vi "New_GraphDisp.vi"() -> ()   [LabVIEW 2016, in "PanelSplitForDisplay.lvclass"]
uses:
  PanelSplit/PanelSplitForDisplay.lvclass
  PanelSplit/PanelObject/PanelObject.lvclass
  <vilib>/Utility/error.llb/DialogType.ctl
  PanelSplit/PanelDataNode/PanelDataNode.lvclass
  Architecture/Queue Management/ARC_Queue Create_Single.vi
  Architecture/Queue Management/ARC_Queue Remove Element.vi
  Ctrls/GlobeVaribles.vi
  Architecture/Queue Management/ARC_Queue Insert Element.vi
  Architecture/Queue Management/ARC_Queue Destroy_Single.vi
panel:
  in  "Node*":refnum<data-value>
  out "Waveform Chart":waveform(dbl)(graph)
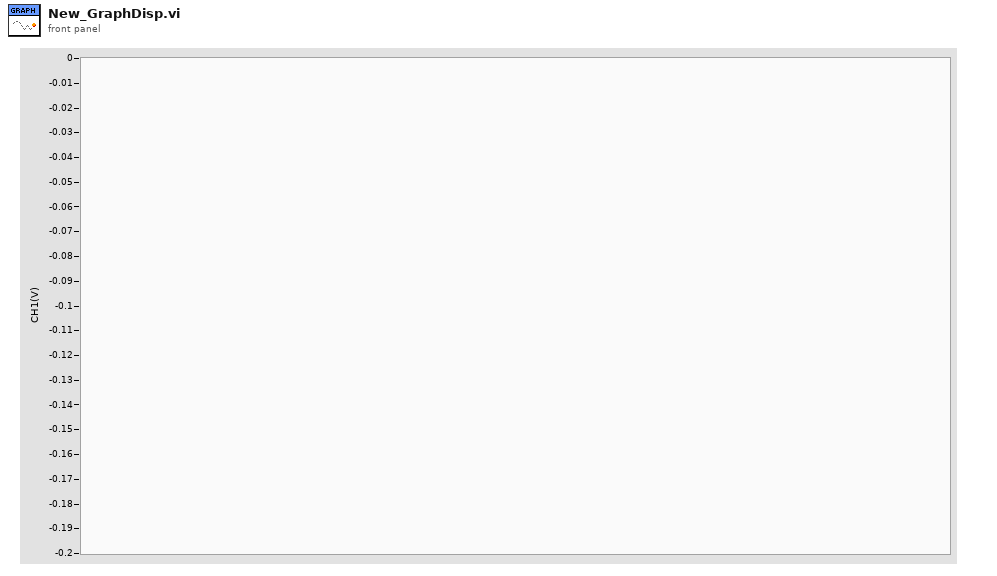
[diagram p1: front panel]
types:
  T1 = cluster{"error":errorcluster, "Event":string, "Data":variant, "Q_Local":string, "Graph":refnum<vi>, "Q_Caller":string}
  T2 = typedef "DialogType.ctl" = u16
  T3 = typedef "LVRectTypeDef.ctl" = cluster{"Left":i16, "Top":i16, "Right":i16, "Bottom":i16}
  T4 = typedef "PanelSplitForDisplay.lvclass/ViValueCtl.ctl" = cluster{"CHTag":string, "GraphProperts":cluster{"YMax":dbl, "YMin":dbl, "ScaleFit":u8}, "CHUnit":string, "CHName":string, "CHValue":string, "CHAlias":string}
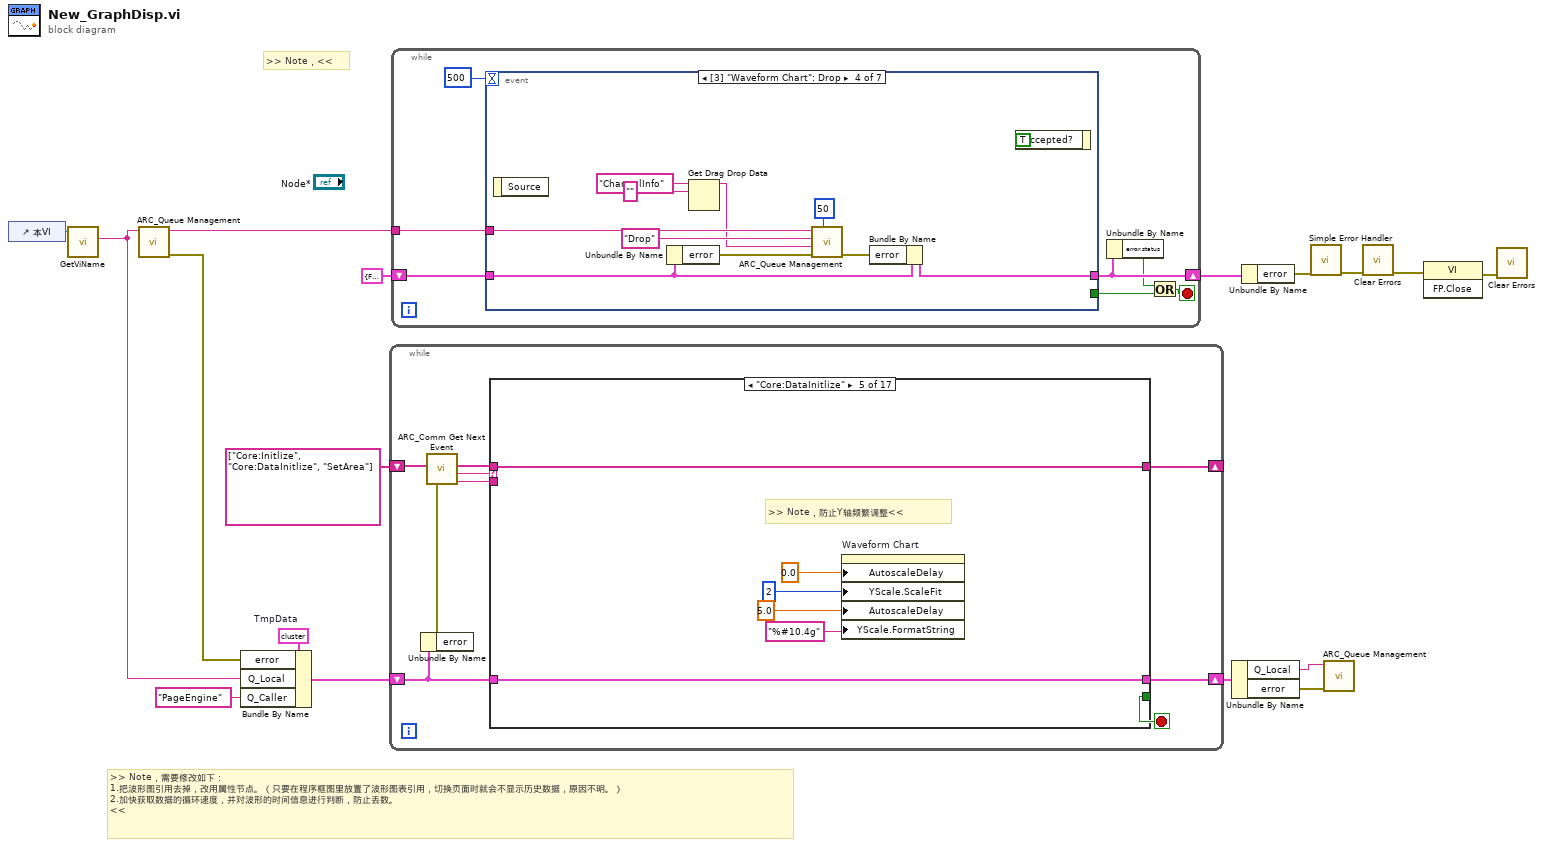
[diagram p0: block diagram]
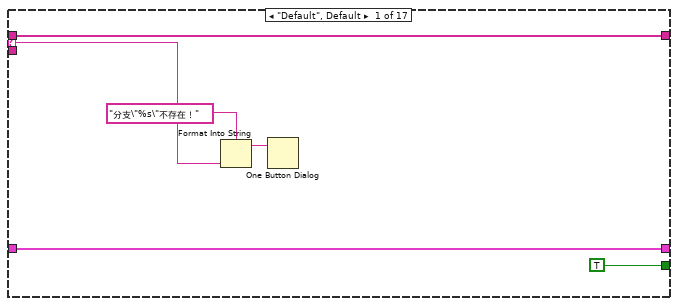
[diagram p2: hidden frame]
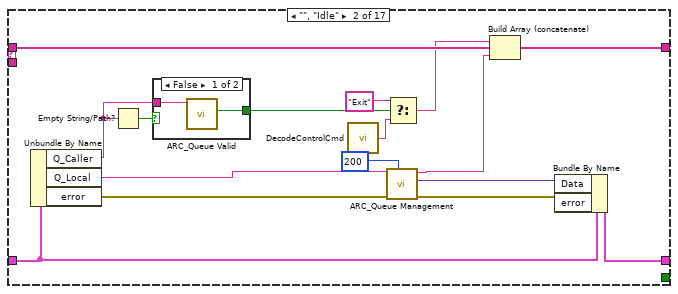
[diagram p3: hidden frame]
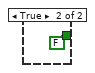
[diagram p4: hidden frame]
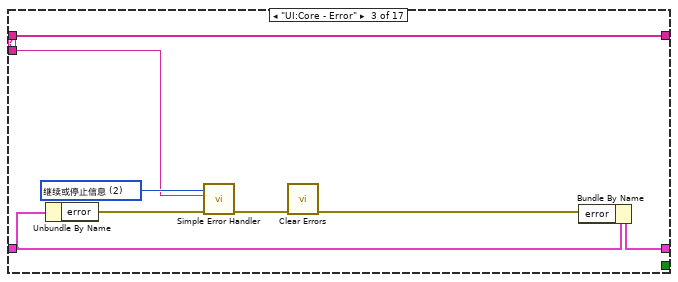
[diagram p5: hidden frame]
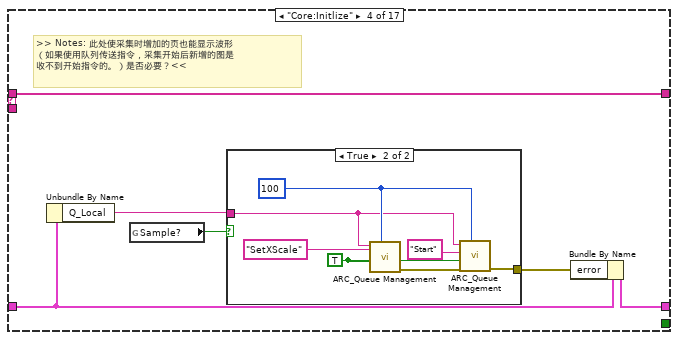
[diagram p6: hidden frame]
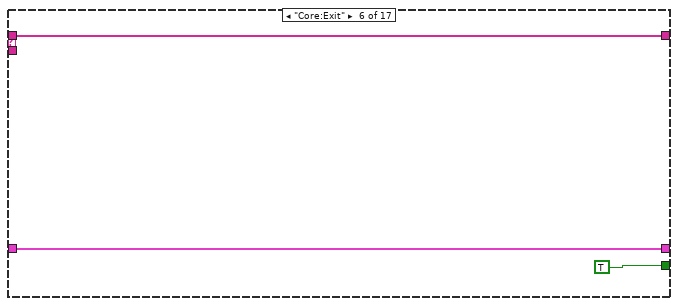
[diagram p8: hidden frame]
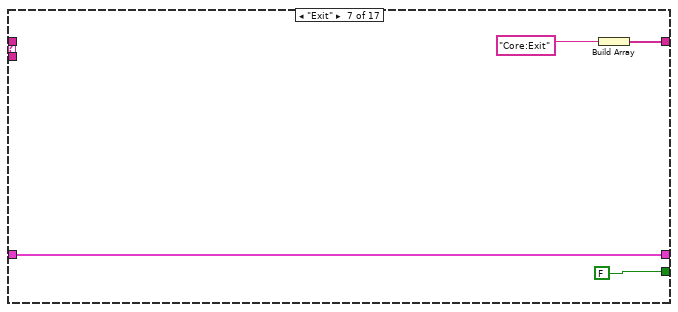
[diagram p9: hidden frame]
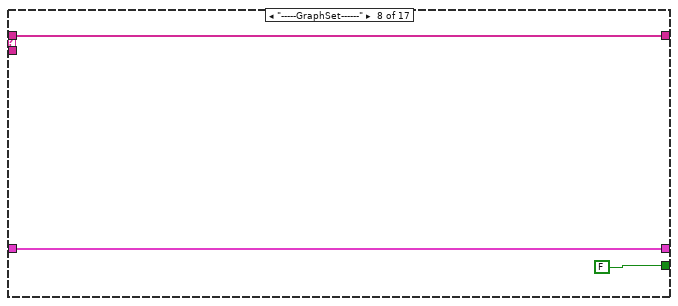
[diagram p10: hidden frame]
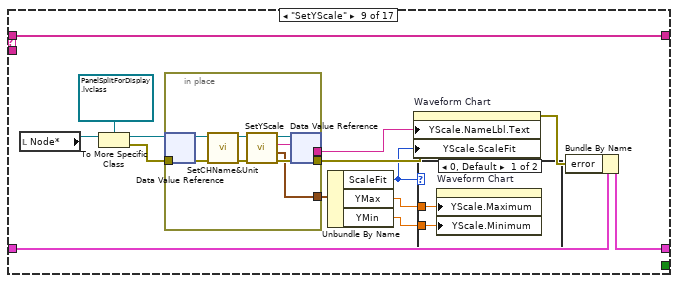
[diagram p11: hidden frame]
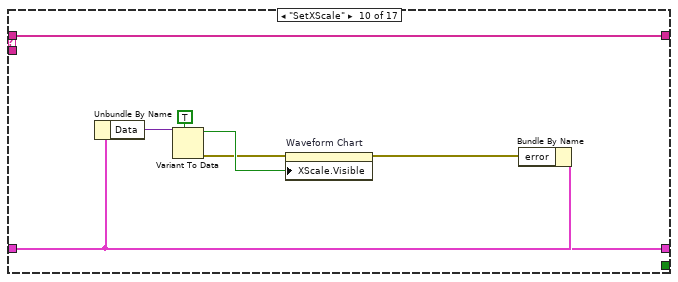
[diagram p13: hidden frame]
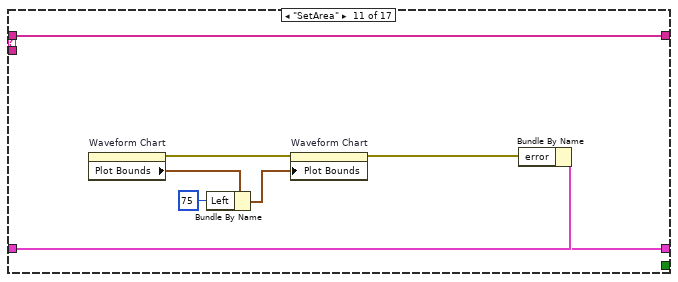
[diagram p14: hidden frame]
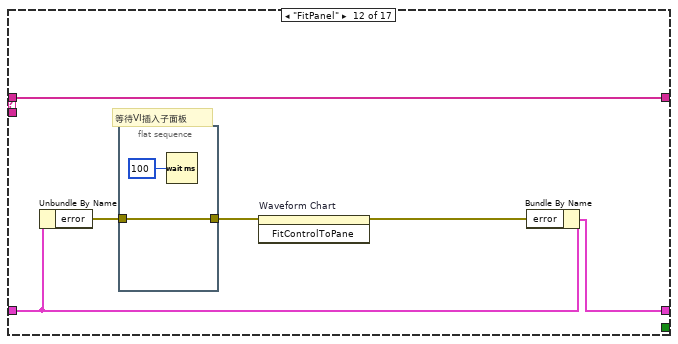
[diagram p15: hidden frame]
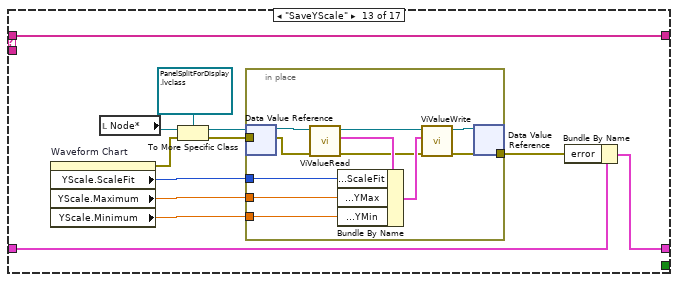
[diagram p16: hidden frame]
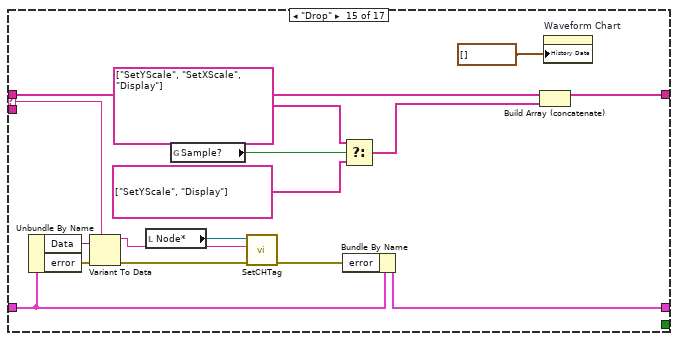
[diagram p18: hidden frame]
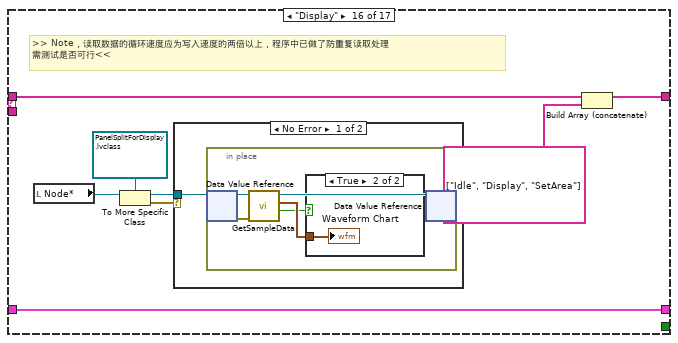
[diagram p19: hidden frame]
diagram:
  w14 = T1 {"error"={"status"=FALSE, "code"=0, "source"=""}, "Event"="", "Data"=variant, "Q_Local"="", "Graph"=refnum, "Q_Caller"=""}  # TmpData
  # ">> Note，<<"
  # ">> Note，需要修改如下：\n1.把波形图引用去掉，改用属性节点。（只要在程序框图里放置了波形图表引用，切换页面时就会不显示历史数据，原因不明。）\n2.加快获取数据的循环速度，并对波形的时间信息进行判断，防止丢数。\n<<"
  n1 = control-ref of="本VI"() -> (w7:refnum<vi>)
  n2 = call "GetViName.vi"("VI*"=w7) -> ("VI Name"=w10:string)  [unwired: 9 in, 1 out]
  n3 = call-poly "ARC_Queue Management.vi"("Queue Name"=w10) -> ("error out"=w11:errorcluster)  [unwired: 8 in, 2 out]
  n4 = Bundle By Name(cluster=w14, "error"=w11, "Q_Local"=w10, "Q_Caller"="PageEngine") -> (w13:T1)
  n5 = while {
    shift-right: [w21] -> w15
    shift-left: w13 -> [w22]
    shift-right: [w20] -> _
    shift-left: string[] ["Core:Initlize", "Core:DataInitlize", "SetArea"] ("event queue out") -> [w19]
    stop <- w24 stop-if-true
    n6 = Unbundle By Name(w22) -> ("error"=w23:errorcluster)
    n7 = call "ARC_Comm Get Next Event.vi"("error in (no error)"=w23, "event queue in"=w19) -> ("prev event"=w25:string, "next event"=w17:string, "event queue out"=w18:string[])  [unwired: 4 in]
    n8 = case shown="\"Core:DataInitlize\"" w17 {
      selector: w17 -> [w29 _ _ _ _ _ _ _ _ _ _ _ _ _ w164 _ _]
      tunnel: w18 -> [w30 w36 w58 w59 w77 w78 _ w85 w101 w119 w127 w133 w147 w159 w175 w179 w192]
      tunnel: w25 -> [_ _ w51 _ _ _ _ _ _ _ _ _ _ _ _ _ _]
      tunnel: [TRUE _ _ _ _ TRUE FALSE FALSE _ _ _ _ _ _ _ _ _] -> w24
      tunnel: w22 -> [w31 w44 w54 w63 w76 w79 w83 w86 w94 w116 w126 w129 w138 w160 w172 w184 w193]
      tunnel: [w31 w46 w53 w64 w76 w79 w83 w86 w93 w115 w125 w131 w137 w160 w162 w184 w193] -> w21
      tunnel: [w30 w35 w58 w59 w77 w78 w81 w85 w101 w119 w127 w133 w147 w159 w174 w178 w192] -> w20
      frame "Default", Default {
        n9 = Format Into String(format string="分支\"%s\"不存在！" ("格式字符串"), w29) -> (resulting string=w28:string)  [unwired: 2 in, 1 out]
        n10 = One Button Dialog(message=w28) -> ()  [unwired: 1 in, 1 out]
      }
      frame "", "Idle" {
        n11 = Unbundle By Name(w44) -> ("Q_Caller"=w39:string, "Q_Local"=w43:string, "error"=w37:errorcluster)
        n12 = Empty String/Path?(string/path=w39) -> (empty?=w40:bool)
        n13 = case shown="False" w40 {
          tunnel: [w48 FALSE ("Not Exist?")] -> w38
          tunnel: w39 -> [w49 _]
          frame False {
            n14 = call "ARC_Queue Valid.vi"("Queue Name(unamed)"=w49) -> ("Not Exist?"=w48:bool)  [unwired: 8 in, 2 out]
          }
          frame True {
          }
        }
        n15 = call "DecodeControlCmd.vi"() -> ("Command"=w41:string)
        n16 = call-poly "ARC_Queue Management.vi"("Time out(-1)_queue out"=200 ("Time out(-1)"), "error in (no error)"=w37, "Queue Name(unamed)"=w43) -> ("error out"=w47:errorcluster, "Data"=w45:variant, "Event"=w33:string)  [unwired: 5 in, 1 out]
        n17 = Select(t="Exit" ("Event"), s=w38, f=w41) -> (s? t:f=w34:string)
        n18 = Build Array (concatenate)(w34, w36, w33) -> (w35:string[])
        n19 = Bundle By Name(cluster=w44, "Data"=w45, "error"=w47) -> (w46:T1)
      }
      frame "UI:Core - Error" {
        w52 = T2 2 items=["无对话框", "确定信息", "继续或停止信息", "确定信息＋警告", "继续/停止+警告"] ("type of dialog (OK msg:1)")
        n20 = Unbundle By Name(w54) -> ("error"=w55:errorcluster)
        n21 = call <vilib>:"Simple Error Handler.vi"("error source (\" \")"=w51, "type of dialog (OK msg:1)"=w52, "error in (no error)"=w55) -> ("error out"=w56:errorcluster)  [unwired: 2 in, 4 out]
        n22 = call <vilib>:"Clear Errors.vi"("error in (no error)"=w56) -> ("error out"=w57:errorcluster)  [unwired: 5 in, 1 out]
        n23 = Bundle By Name(cluster=w54, "error"=w57) -> (w53:T1)
      }
      frame "Core:Initlize" {
        # ">> Notes: 此处使采集时增加的页也能显示波形\n（如果使用队列传送指令，采集开始后新增的图是\n收不到开始指令的。）是否必要？<<"
        n24 = Unbundle By Name(w63) -> ("Q_Local"=w62:string)
        n25 = global read "GlobeVaribles.vi" "Sample?"() -> (w60:bool)
        n26 = case shown="True" w60 {
          tunnel: w62 -> [_ w67]
          tunnel: [_ w69] -> w61
          frame False {
          }
          frame True {
            w68 = 100 ("Time out(-1)_queue in")
            w65 = TRUE
            n27 = call-poly "ARC_Queue Management.vi"("Time out(-1)_queue in"=w68, "Data"=w65, "Event"="SetXScale", "Queue Name(unamed)"=w67) -> ("error out"=w70:errorcluster)  [unwired: 6 in, 1 out]
            n28 = call-poly "ARC_Queue Management.vi"("Time out(-1)_queue in"=w68, "error in (no error)"=w70, "Data"=w65, "Event"="Start", "Queue Name(unamed)"=w67) -> ("error out"=w69:errorcluster)  [unwired: 5 in, 1 out]
          }
        }
        n29 = Bundle By Name(cluster=w63, "error"=w61) -> (w64:T1)
      }
      frame "Core:DataInitlize" {
        # ">> Note，防止Y轴频繁调整<<"
        n30 = property on="Waveform Chart" class="WFChart (strict)"("AutoscaleDelay"=sgl 0.0 ("自动调整标尺延迟"), "YScale.ScaleFit"=u8 2 ("Y标尺.标尺调节"), "AutoscaleDelay"=sgl 5.0 ("自动调整标尺延迟"), "YScale.FormatString"="%#10.4g" ("Y标尺.格式字符串")) -> ()  [unwired: 2 in, 2 out]
      }
      frame "Core:Exit" {
      }
      frame "Exit" {
        n31 = Build Array("Core:Exit" ("Remaining States")) -> (w81:string[])
      }
      frame "-----GraphSet------" {
      }
      frame "SetYScale" {
        n32 = local read "Node*"() -> (w100:refnum<data-value>)
        n33 = To More Specific Class(target class=refnum<data-value> refnum ("数据值引用"), reference=w100) -> (specific class reference=w99:refnum<data-value>, error out=w97:errorcluster)  [unwired: 1 in]
        n34 = in-place {
          in-place-border: w97 -> [w106]
          in-place-border: [w110] -> w96
          in-place-border: [w109] -> w95
          in-place-border: [w104] -> w92
          n35 = in-place-dvr #1(w99) -> (w108:refnum<class "PanelSplitForDisplay.lvclass">)  [unwired: 1 out]
          n36 = call "SetCHName&Unit.vi"("error in (no error)"=w106, "PanelSplitForDisplay 输入"=w108) -> ("error out"=w105:errorcluster, "PanelSplitForDisplay 输出"=w107:refnum<class "PanelSplitForDisplay.lvclass">)  [unwired: 8 in]
          n37 = call "SetYScale.vi"("error in"=w105, "PanelSplitForDisplay 输入"=w107) -> ("error out"=w109:errorcluster, "GraphProperts"=w104:cluster{"YMax":dbl, "YMin":dbl, "ScaleFit":u8}, "YLable"=w110:string, "PanelSplitForDisplay 输出"=w111:refnum<class "PanelSplitForDisplay.lvclass">)  [unwired: 6 in]
          n38 = in-place-dvr #1(w111) -> ()  [unwired: 2 out]
        }
        n39 = Unbundle By Name(w92) -> ("ScaleFit"=w91:u8, "YMax"=w90:dbl, "YMin"=w89:dbl)
        n40 = property on="Waveform Chart" class="WFChart (strict)"(error in=w95, "YScale.NameLbl.Text"=w96, "YScale.ScaleFit"=w91) -> (error out=w88:errorcluster)  [unwired: 1 in, 1 out]
        n41 = case shown="0, Default" w91 {
          tunnel: w90 -> [w103 _]
          tunnel: w89 -> [w102 _]
          frame 0, Default {
            n42 = property on="Waveform Chart" class="WFChart (strict)"("YScale.Maximum"=w103, "YScale.Minimum"=w102) -> ()  [unwired: 2 in, 2 out]
          }
          frame 2 {
          }
        }
        n43 = Bundle By Name(cluster=w94, "error"=w88) -> (w93:T1)
      }
      frame "SetXScale" {
        n44 = Unbundle By Name(w116) -> ("Data"=w117:variant)
        n45 = Variant To Data(type=TRUE ("X标尺.可见"), Variant=w117) -> (data=w114:bool, error out=w113:errorcluster)  [unwired: 1 in]
        n46 = property on="Waveform Chart" class="WFChart (strict)"(error in=w113, "XScale.Visible"=w114) -> (error out=w112:errorcluster)  [unwired: 1 in, 1 out]
        n47 = Bundle By Name(cluster=w116, "error"=w112) -> (w115:T1)
      }
      frame "SetArea" {
        n48 = property on="Waveform Chart" class="WFChart (strict)"() -> (error out=w120:errorcluster, "Plot Bounds"=w123:T3)  [unwired: 2 in, 1 out]
        n49 = Bundle By Name(cluster=w123, "Left"=i16 75 ("left")) -> (w122:T3)
        n50 = property on="Waveform Chart" class="WFChart (strict)"(error in=w120, "Plot Bounds"=w122) -> (error out=w124:errorcluster)  [unwired: 1 in, 1 out]
        n51 = Bundle By Name(cluster=w126, "error"=w124) -> (w125:T1)
      }
      frame "FitPanel" {
        # "等待VI插入子面板"
        n52 = Unbundle By Name(w129) -> ("error"=w128:errorcluster)
        n53 = flat-sequence {
          tunnel: [w134] -> w130
          tunnel: w128 -> [w134]
          frame #0 {
            n54 = Wait (ms)(milliseconds to wait=u32 100 ("等待时间（毫秒）")) -> ()  [unwired: 1 out]
          }
        }
        n55 = invoke on="Waveform Chart" class="WFChart (严格)" method="FitControlToPane"(error in=w130) -> (error out=w132:errorcluster)  [unwired: 2 in, 2 out]
        n56 = Bundle By Name(cluster=w129, "error"=w132) -> (w131:T1)
      }
      frame "SaveYScale" {
        n57 = property on="Waveform Chart" class="WFChart (strict)"() -> (error out=w136:errorcluster, "YScale.ScaleFit"=w142:u8, "YScale.Maximum"=w141:dbl, "YScale.Minimum"=w140:dbl)  [unwired: 2 in, 1 out]
        n58 = local read "Node*"() -> (w146:refnum<data-value>)
        n59 = To More Specific Class(target class=refnum<data-value> refnum ("数据值引用"), reference=w146, error in=w136) -> (specific class reference=w143:refnum<data-value>, error out=w144:errorcluster)
        n60 = in-place {
          in-place-border: w144 -> [w150]
          in-place-border: w142 -> [w153]
          in-place-border: w141 -> [w152]
          in-place-border: w140 -> [w151]
          in-place-border: [w148] -> w139
          n61 = in-place-dvr #2(w143) -> (w158:refnum<class "PanelSplitForDisplay.lvclass">)  [unwired: 1 out]
          n62 = call "ViValueRead.vi"("error in (no error)"=w150, "PanelSplitForDisplay 输入"=w158) -> ("error out"=w149:errorcluster, "ViValue"=w155:T4, "PanelSplitForDisplay 输出"=w157:refnum<class "PanelSplitForDisplay.lvclass">)  [unwired: 7 in]
          n63 = Bundle By Name(cluster=w155, "GraphProperts.ScaleFit"=w153, "GraphProperts.YMax"=w152, "GraphProperts.YMin"=w151) -> (w154:T4)
          n64 = call "ViValueWrite.vi"("error in (no error)"=w149, "ViValue"=w154, "PanelSplitForDisplay 输入"=w157) -> ("error out"=w148:errorcluster, "PanelSplitForDisplay 输出"=w156:refnum<class "PanelSplitForDisplay.lvclass">)  [unwired: 7 in]
          n65 = in-place-dvr #2(w156) -> ()  [unwired: 2 out]
        }
        n66 = Bundle By Name(cluster=w138, "error"=w139) -> (w137:T1)
      }
      frame "----------------------" {
      }
      frame "Drop" {
        n67 = Unbundle By Name(w172) -> ("Data"=w165:variant, "error"=w167:errorcluster)
        n68 = Variant To Data(error in=w167, type=w164, Variant=w165) -> (data=w163:string, error out=w166:errorcluster)
        n69 = local read "Node*"() -> (w173:refnum<data-value>)
        n70 = global read "GlobeVaribles.vi" "Sample?"() -> (w171:bool)
        n71 = call "SetCHTag.vi"("error in (no error)"=w166, "ChannelTag"=w163, "Node*"=w173) -> ("error out"=w161:errorcluster)  [unwired: 8 in]
        n72 = Bundle By Name(cluster=w172, "error"=w161) -> (w162:T1)
        n73 = Select(t=string[] ["SetYScale", "SetXScale", "Display"] ("event queue out"), s=w171, f=string[] ["SetYScale", "Display"] ("event queue out")) -> (s? t:f=w168:string[])
        n74 = Build Array (concatenate)(w175, w168) -> (w174:string[])
        n75 = property on="Waveform Chart" class="WFChart (strict)"("History Data"=waveform(dbl)[] [] ("历史数据")) -> ()  [unwired: 2 in, 2 out]
      }
      frame "Display" {
        # ">> Note，读取数据的循环速度应为写入速度的两倍以上，程序中已做了防重复读取处理\n需测试是否可行<<"
        n76 = local read "Node*"() -> (w183:refnum<data-value>)
        n77 = To More Specific Class(target class=refnum<data-value> refnum ("数据值引用"), reference=w183) -> (specific class reference=w182:refnum<data-value>, error out=w180:errorcluster)  [unwired: 1 in]
        n78 = case shown="No Error" w180 {
          tunnel: w182 -> [w185 _]
          frame No Error {
            n79 = in-place {
              n80 = in-place-dvr #3(w185) -> (w190:refnum<class "PanelSplitForDisplay.lvclass">, w187:errorcluster)
              n81 = call "GetSampleData.vi"("error in"=w187, "PanelSplitForDisplay.lvclass"=w190) -> ("Display?"=w186:bool, "signal out"=w188:waveform(dbl), "PanelSplitForDisplay.lvclass 2"=w189:refnum<class "PanelSplitForDisplay.lvclass">)  [unwired: 3 in, 2 out]
              n82 = case shown="True" w186 {
                tunnel: w188 -> [_ w191]
                frame False {
                }
                frame True {
                  "Waveform Chart" <- w191
                }
              }
              n83 = in-place-dvr #3(w189) -> ()  [unwired: 2 out]
            }
          }
          frame Error {
          }
        }
        n84 = Build Array (concatenate)(w179, string[] ["Idle", "Display", "SetArea"] ("event queue out")) -> (w178:string[])
      }
      frame "Stop" {
      }
    }
  }
  n85 = while {
    tunnel: w10 -> [w200]
    shift-right: [w195] -> w8
    shift-left: cluster{"Float?":bool, "error":errorcluster} {"Float?"=FALSE, "error"={"status"=FALSE, "code"=0, "source"=""}} -> [w199]
    stop <- w197 stop-if-true
    n86 = event shown="[3] \"Waveform Chart\": Drop" {
      selector: _ -> [_ _ _ _ _ _ _]
      dyn-events: _ -> [_ _ _ _ _ _ _]
      timeout: 500 -> [_ _ _ _ _ _ _]
      tunnel: [w201 _ _ _ _ _ FALSE] -> w198
      tunnel: w200 -> [w204 _ w218 w259 _ w266 _]
      tunnel: w199 -> [w202 w211 w220 w257 w262 w267 w270]
      tunnel: [w202 w211 w219 w255 w262 w267 w269] -> w195
      event Timeout {
        n87 = event-data() -> ()  [unwired: 1 in, 2 out]
        n88 = Unbundle By Name(w202) -> ("error"=w203:errorcluster)
        n89 = call-poly "ARC_Queue Management.vi"("error in"=w203, "Queue Name"=w204) -> ("Created New?"=w201:bool)  [unwired: 7 in, 2 out]
      }
      event "Waveform Chart": Shortcut Menu Activation? {
        w205 = string[] ["显示", "隐藏"] ("f")
        n90 = event-data() -> ("MenuRef"=w215:refnum<k9>)  [unwired: 1 in]
        n91 = Unbundle By Name(w211) -> ("Float?"=w210:bool)
        n92 = Not(x=w210) -> (.not. x?=w209:bool)
        n93 = Select(t=string[] ["删除", "浮动", "时间轴", "自动调整Y标尺"] ("项名称"), s=w209, f=string[] ["返回", "时间轴"]) -> (s? t:f=w213:string[])
        n94 = Delete Menu Items(9:w215) -> (0:w216:errorcluster, 3:w217:refnum<k9>)  [unwired: 3 in]
        n95 = Insert Menu Items(6:w216, 7:w213, 8:w213, 9:w217) -> (0:w207:errorcluster, 3:w208:refnum<k9>)  [unwired: 2 in, 1 out]
        n96 = Insert Menu Items(5:"时间轴", 6:w207, 7:w205, 8:w205, 9:w208) -> ()  [unwired: 1 in, 3 out]
        n97 = event-data() -> ()  [unwired: 2 in, 1 out]
      }
      event "Waveform Chart": Shortcut Menu Selection (User) {
        n98 = event-data() -> ("ItemTag"=w222:string)  [unwired: 1 in]
        n99 = local read "Node*"() -> (w223:refnum<data-value>)
        n100 = To More Specific Class(target class=refnum<data-value> refnum ("Node*"), reference=w223) -> (specific class reference=w221:refnum<data-value>)  [unwired: 1 in, 1 out]
        n101 = case shown="\"浮动\"" w222 {
          tunnel: w221 -> [_ w227 w231 w238 _ _ _ _]
          tunnel: w220 -> [w225 w226 w230 w237 w243 w245 w246 w250]
          tunnel: [w225 w226 w229 w235 w243 w245 w246 w250] -> w219
          tunnel: w218 -> [_ _ _ _ _ _ _ w247]
          frame "假", Default {
          }
          frame "删除" {
            n102 = call "Q_Delete.vi"("ChildNode*"=w227) -> ()  [unwired: 10 in, 1 out]
          }
          frame "浮动" {
            n103 = in-place {
              n104 = in-place-dvr #4(w231) -> (w234:refnum<class "PanelDataNode.lvclass">, w232:errorcluster)
              n105 = call "RefreshPanel.vi"("error in (no error)"=w232, "PanelDataNode 输入"=w234) -> ("PanelDataNode 输出"=w233:refnum<class "PanelDataNode.lvclass">)  [unwired: 8 in, 1 out]
              n106 = in-place-dvr #4(w233) -> ()  [unwired: 2 out]
            }
            n107 = Bundle By Name(cluster=w230, "Float?"=TRUE) -> (w229:cluster{"Float?":bool, "error":errorcluster})
          }
          frame "返回" {
            n108 = in-place {
              n109 = in-place-dvr #5(w238) -> (w241:refnum<class "PanelDataNode.lvclass">, w239:errorcluster)
              n110 = call "BackToPanel.vi"("error in (no error)"=w239, "PanelDataNode 输入"=w241) -> ("PanelDataNode 输出"=w240:refnum<class "PanelDataNode.lvclass">)  [unwired: 8 in, 1 out]
              n111 = in-place-dvr #5(w240) -> ()  [unwired: 2 out]
            }
            n112 = Bundle By Name(cluster=w237, "Float?"=FALSE) -> (w235:cluster{"Float?":bool, "error":errorcluster})
          }
          frame "显示" {
            n113 = property on="Waveform Chart" class="WFChart (strict)"("XScale.Visible"=TRUE ("X标尺.可见")) -> ()  [unwired: 2 in, 2 out]
          }
          frame "隐藏" {
            n114 = property on="Waveform Chart" class="WFChart (strict)"("XScale.Visible"=FALSE ("X标尺.可见")) -> ()  [unwired: 2 in, 2 out]
          }
          frame "Fit" {
            n115 = invoke on="Waveform Chart" class="WFChart (严格)" method="FitControlToPane"() -> ()  [unwired: 3 in, 3 out]
          }
          frame "自动调整Y标尺" {
            n116 = property on="Waveform Chart" class="WFChart (strict)"("YScale.ScaleFit"=u8 2 ("Y标尺.标尺调节")) -> ()  [unwired: 2 in, 2 out]
            n117 = call-poly "ARC_Queue Management.vi"("Event"="SaveYScale", "Queue Name(unamed)"=w247) -> ()  [unwired: 8 in, 2 out]
          }
        }
      }
      event "Waveform Chart": Drop {
        n118 = event-data() -> ()  [unwired: 1 in, 1 out]
        n119 = Unbundle By Name(w257) -> ("error"=w256:errorcluster)
        n120 = Get Drag Drop Data(8:"", 9:"ChannelInfo" ("数据名称")) -> (3:w251:string)  [unwired: 1 in, 1 out]
        n121 = call-poly "ARC_Queue Management.vi"("Time out(-1)_queue in"=50, "error in (no error)"=w256, "Data"=w251, "Event"="Drop", "Queue Name(unamed)"=w259) -> ("error out"=w254:errorcluster)  [unwired: 5 in, 1 out]
        n122 = Bundle By Name(cluster=w257, "error"=w254) -> (w255:cluster{"Float?":bool, "error":errorcluster})
        n123 = event-data("Accepted?"=TRUE ("接受？")) -> ()  [unwired: 1 in, 1 out]
      }
      event "Waveform Chart": Drag Enter {
        n124 = event-data() -> ()  [unwired: 1 in, 1 out]
        n125 = event-data("Accepted?"=TRUE ("接受？")) -> ()  [unwired: 1 in, 1 out]
      }
      event "Waveform Chart": Scale Range Change {
        n126 = event-data() -> ()  [unwired: 1 in, 2 out]
        n127 = property on="Waveform Chart" class="WFChart (strict)"("YScale.ScaleFit"=u8 0 ("Y标尺.标尺调节")) -> ()  [unwired: 2 in, 2 out]
        n128 = call-poly "ARC_Queue Management.vi"("Event"="SetArea\nSaveYScale", "Queue Name(unamed)"=w266) -> ()  [unwired: 8 in, 2 out]
      }
      event Panel Close? {
        n129 = event-data() -> ()  [unwired: 1 in, 1 out]
        n130 = local read "Node*"() -> (w271:refnum<data-value>)
        n131 = To More Specific Class(target class=refnum<data-value> refnum ("Node*"), reference=w271) -> (specific class reference=w273:refnum<data-value>, error out=w272:errorcluster)  [unwired: 1 in]
        n132 = case shown="No Error" w272 {
          selector: w272 -> [w278 w284]
          tunnel: w273 -> [w279 _]
          tunnel: [w277 w284] -> _
          frame No Error {
            n133 = in-place {
              in-place-border: w278 -> [w281]
              in-place-border: [w280] -> w277
              n134 = in-place-dvr #6(w279) -> (w283:refnum<class "PanelDataNode.lvclass">)  [unwired: 1 out]
              n135 = call "BackToPanel.vi"("error in (no error)"=w281, "PanelDataNode 输入"=w283) -> ("error out"=w280:errorcluster, "PanelDataNode 输出"=w282:refnum<class "PanelDataNode.lvclass">)  [unwired: 8 in]
              n136 = in-place-dvr #6(w282) -> ()  [unwired: 2 out]
            }
          }
          frame Error {
          }
        }
        n137 = Bundle By Name(cluster=w270, "Float?"=FALSE) -> (w269:cluster{"Float?":bool, "error":errorcluster})
        n138 = event-data("Discard?"=TRUE ("放弃？")) -> ()  [unwired: 1 in, 1 out]
      }
    }
    n139 = Unbundle By Name(w195) -> ("error.status"=w194:bool)
    n140 = Or(x=w194, y=w198) -> (x .or. y?=w197:bool)
  }
  n141 = Unbundle By Name(w15) -> ("Q_Local"=w12:string, "error"=w16:errorcluster)
  n142 = Unbundle By Name(w8) -> ("error"=w5:errorcluster)
  n143 = call <vilib>:"Simple Error Handler.vi"("error in (no error)"=w5) -> ("error out"=w3:errorcluster)  [unwired: 4 in, 4 out]
  n144 = call-poly "ARC_Queue Management.vi"("error in (no error)"=w16, "Queue Name(unamed)"=w12) -> ()  [unwired: 7 in, 3 out]
  n145 = call <vilib>:"Clear Errors.vi"("error in (no error)"=w3) -> ("error out"=w2:errorcluster)  [unwired: 5 in, 1 out]
  n146 = invoke class="VI" method="FP.Close"(error in=w2) -> (error out=w4:errorcluster)  [unwired: 2 in, 2 out]
  n147 = call <vilib>:"Clear Errors.vi"("error in (no error)"=w4) -> ()  [unwired: 5 in, 2 out]
